vi "FE and FF Frame Error data Show.vi"(8 "error in (no error)":errorcluster, 10 "Report Data":T1, 11 "Error Log in":refnum<class "Error Log.lvclass">) -> (0 "error out":errorcluster, 3 "Error Log out":refnum<class "Error Log.lvclass">)   [LabVIEW 2023, in "Data Analysis.lvlib" / "Error Log.lvlib" / "Error Log.lvclass"]
uses:
  Error Log.lvclass
  Error Log.lvclass/Error Log.ctl
  HardwareAbstractionLayer_LVOOP/Database/Database.lvclass
  Data Analysis.lvlib
panel:
  in  "FF FRAME":i32(listbox)
  in  "FE FRAME":i32(listbox)
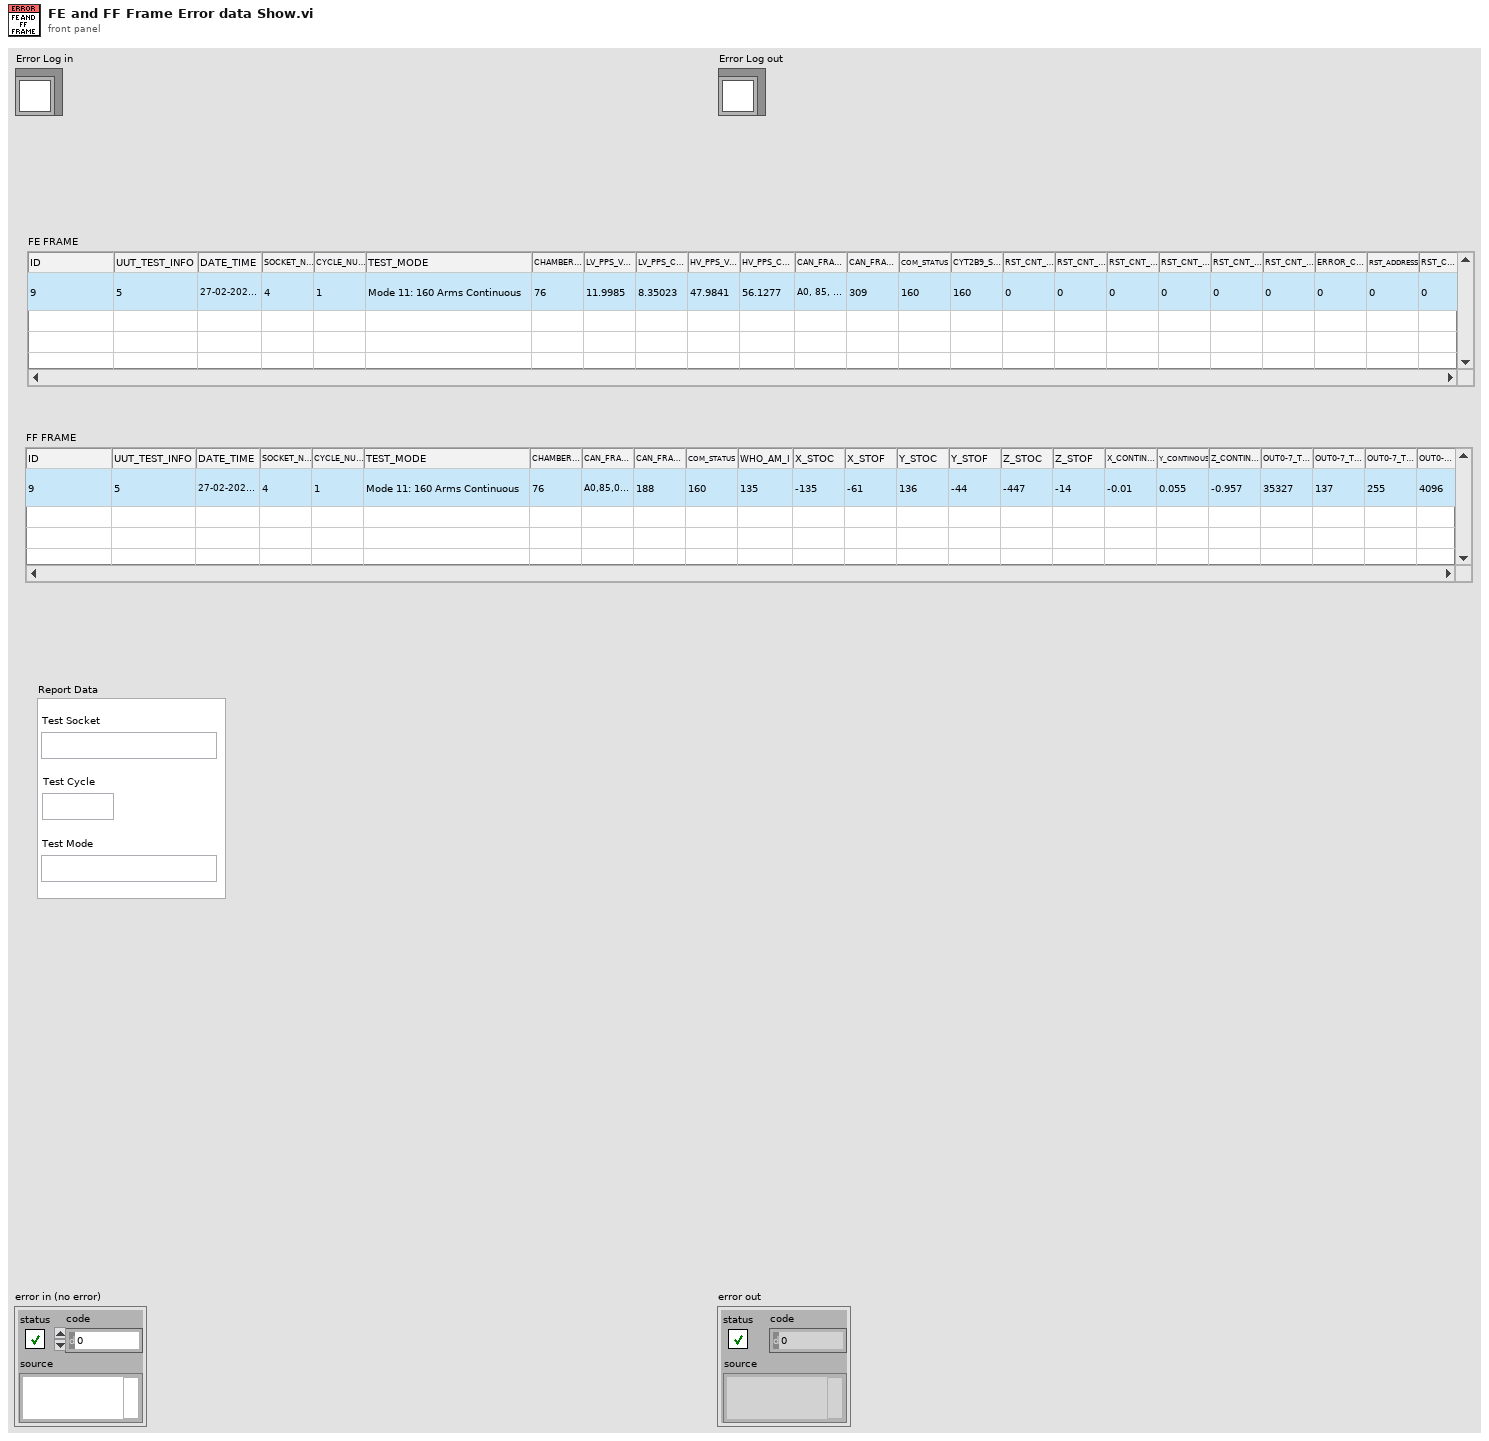
[diagram p1: front panel]
types:
  T1 = cluster{"Test Socket":string, "Test Cycle":string, "Test Mode":string}
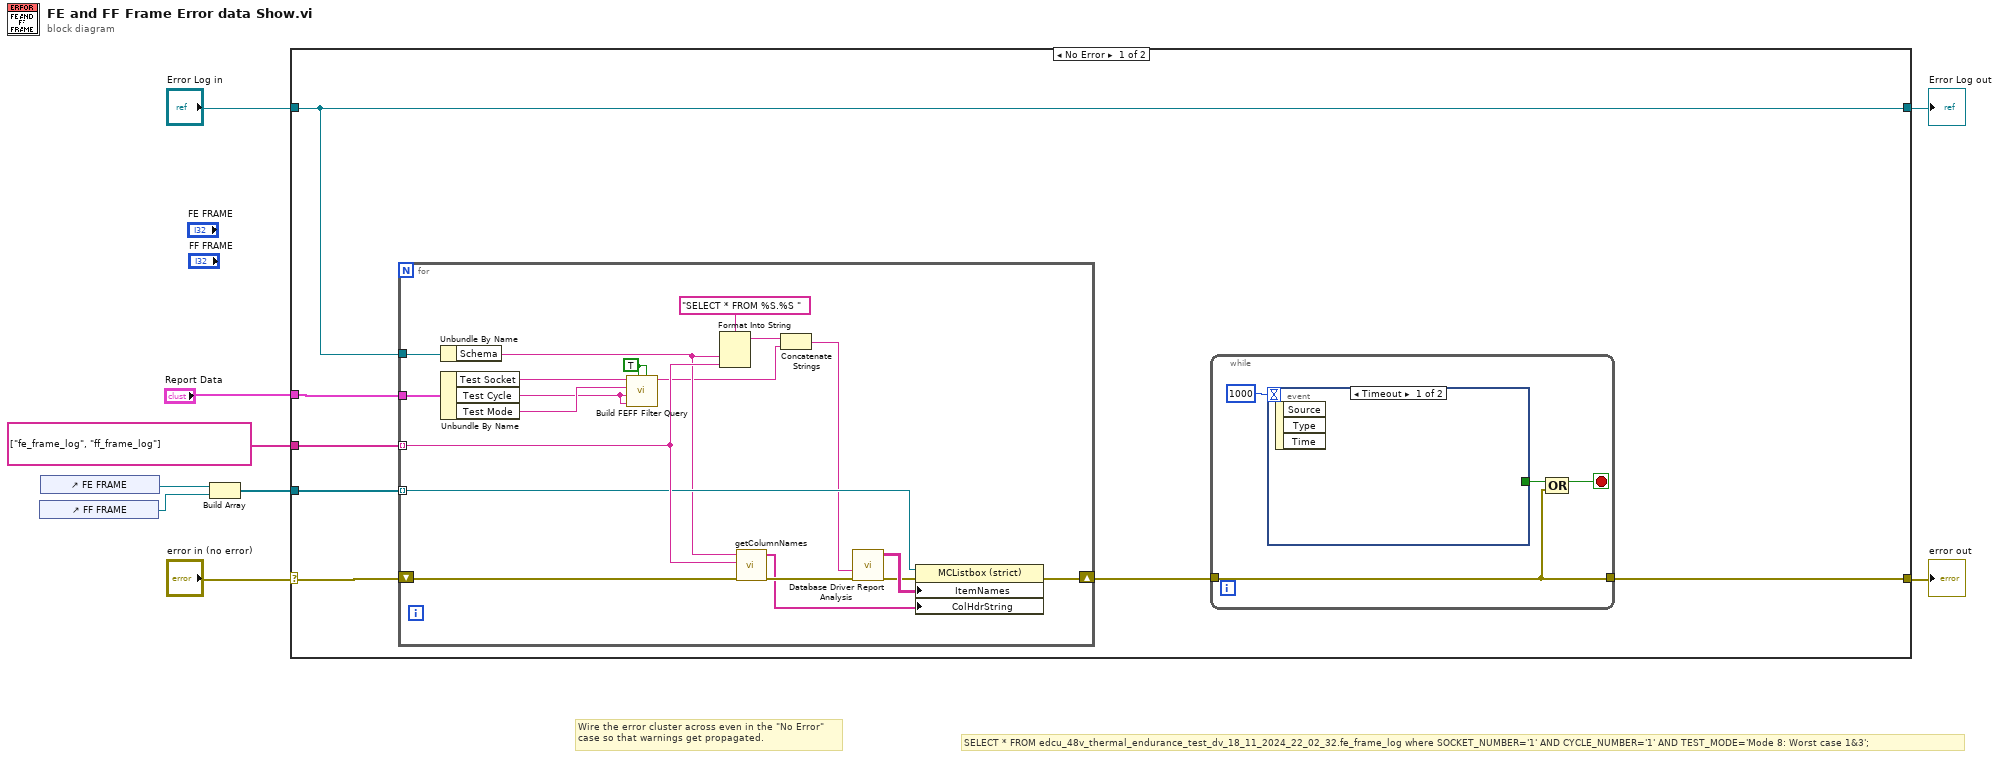
[diagram p0: block diagram]
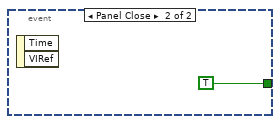
[diagram p2: hidden frame]
diagram:
  # "SELECT * FROM edcu_48v_thermal_endurance_test_dv_18_11_2024_22_02_32.fe_frame_log where SOCKET_NUMBER='1' AND CYCLE_NUMBER='1' AND TEST_MODE='Mode 8: Worst case 1&3';"
  # "Wire the error cluster across even in the \"No Error\"\ncase so that warnings get propagated."
  n1 = control-ref of="FF FRAME"() -> (w1:refnum<vi>)
  n2 = control-ref of="FE FRAME"() -> (w3:refnum<vi>)
  n3 = Build Array(w3, w1) -> (w2:refnum<vi>[])
  n4 = case shown="No Error" "error in (no error)" {
    selector: "error in (no error)" -> [w13 w42]
    tunnel: [w15 w42] -> w8
    tunnel: [w16 w41] -> w6
    tunnel: "Error Log in" -> [w16 w41]
    tunnel: "Report Data" -> [w14 _]
    tunnel: string[] ["fe_frame_log", "ff_frame_log"] -> [w11 _]
    tunnel: w2 -> [w10 _]
    frame No Error {
      n5 = for {
        tunnel: w16 -> [w35]
        tunnel: w14 -> [w33]
        shift-right: [w26] -> w12
        shift-left: w13 -> [w31]
        tunnel: w11 -> [w25] mode=indexing
        tunnel: w10 -> [w24] mode=indexing
        w18 = TRUE ("WHERE needed?(Yes)")
        n6 = Unbundle By Name(w35) -> ("Schema"=w23:string)
        n7 = Unbundle By Name(w33) -> ("Test Socket"=w22:string, "Test Cycle"=w17:string, "Test Mode"=w21:string)
        n8 = call "Build FEFF Filter Query.vi"("ORDER BY needed?(Yes)"=w18, "WHERE needed?(Yes)"=w18, "Stop Test Cycle"=w17, "Start Test Cycle"=w17, "Test Mode"=w21, "Test Socket"=w22) -> ("String"=w19:string)  [unwired: 5 in]
        n9 = Format Into String(format string="SELECT * FROM %S.%S ", w23, w25) -> (resulting string=w32:string)  [unwired: 2 in, 1 out]
        n10 = call "getColumnNames.vi"("error in (no error)"=w31, "tableName"=w25, "schema"=w23) -> ("error out"=w30:errorcluster, "columnNames"=w28:string[])  [unwired: 6 in, 1 out]
        n11 = Concatenate Strings(w32, w19) -> (w20:string)
        n12 = call "Database Driver Report Analysis.vi"("error in"=w30, "SQL query"=w20) -> ("error out"=w27:errorcluster, "data"=w29:string[][])  [unwired: 6 in, 2 out]
        n13 = property class="MCListbox (strict)"(reference=w24, error in=w27, "ItemNames"=w29, "ColHdrString"=w28) -> (error out=w26:errorcluster)  [unwired: 1 out]
      }
      n14 = while {
        tunnel: w12 -> [w36]
        tunnel: [w36] -> w15
        stop <- w37 stop-if-true
        n15 = event shown="[0] Timeout" {
          selector: _ -> [_ _]
          dyn-events: _ -> [_ _]
          timeout: 1000 -> [_ _]
          tunnel: [_ TRUE] -> w38
          event Timeout {
            n16 = event-data() -> ()  [unwired: 1 in, 3 out]
          }
          event Panel Close {
            n17 = event-data() -> ()  [unwired: 1 in, 2 out]
          }
        }
        n18 = Compound Arithmetic op=OR(w38, w36) -> (w37:bool)
      }
    }
    frame Error {
    }
  }
  "error out" <- w8
  "Error Log out" <- w6
